vi "Get Named Ranges of Sheet.vi"(8 "error in":errorcluster, 10 "Sheet Name":string, 11 "SpreadsheetDocument":refnum<k24>) -> (0 "error out":errorcluster, 1 "Cells":string[][][](array[string]), 2 "Range Names":string[](array[string]), 3 "SpreadsheetDocument out":refnum<k24>)   [LabVIEW 2021, in "Open Xml.lvlib"]
uses:
  Open Xml.lvlib
  D:/git/Open-Xml-LabVIEW/Source/DocumentFormat.OpenXml.dll
  DocumentFormat.OpenXml.dll
  D:/git/Open-Xml-LabVIEW/Source/DocumentFormat.OpenXml.Framework.dll
  DocumentFormat.OpenXml.Framework.dll
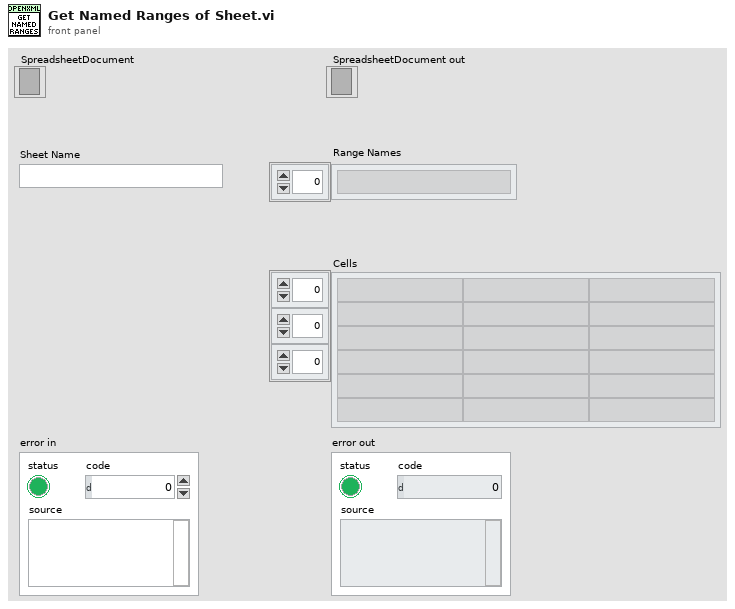
[diagram p1: front panel]
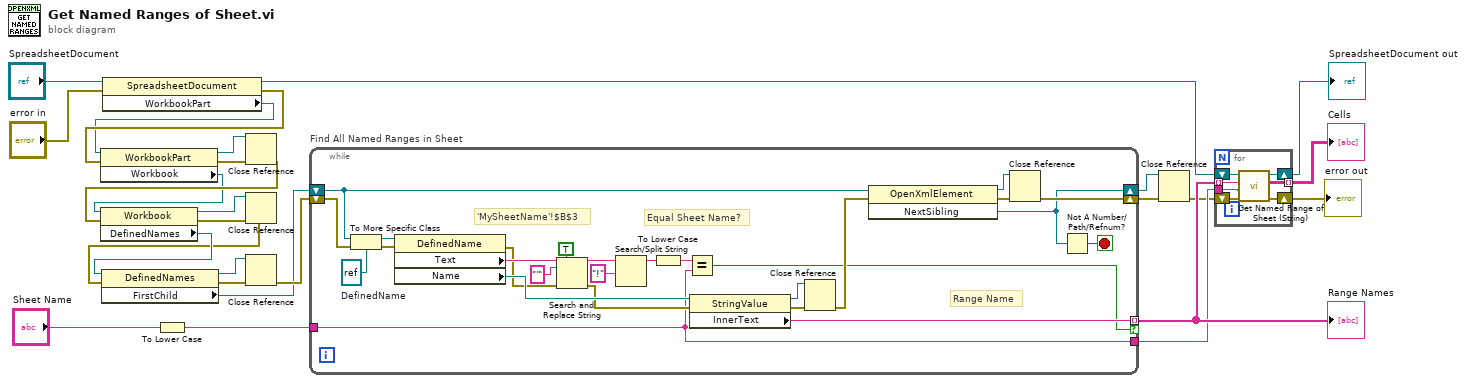
[diagram p0: block diagram]
diagram:
  n1 = property class="SpreadsheetDocument"(reference="SpreadsheetDocument", error in="error in") -> (reference out=w7:refnum<k24>, error out=w14:errorcluster, "WorkbookPart"=w13:refnum<k24>)
  n2 = property class="WorkbookPart"(reference=w13, error in=w14) -> (reference out=w23:refnum<k24>, error out=w25:errorcluster, "Workbook"=w11:refnum<k24>)
  n3 = To Lower Case(string="Sheet Name") -> (all lower case string=w1:string)
  n4 = Close Reference(reference=w23, error in (no error)=w25) -> (error out=w12:errorcluster)
  n5 = property class="Workbook"(reference=w11, error in=w12) -> (reference out=w21:refnum<k24>, error out=w24:errorcluster, "DefinedNames"=w27:refnum<k24>)
  n6 = Close Reference(reference=w21, error in (no error)=w24) -> (error out=w22:errorcluster)
  n7 = property class="DefinedNames"(reference=w27, error in=w22) -> (reference out=w20:refnum<k24>, error out=w26:errorcluster, "FirstChild"=w17:refnum<k24>)
  n8 = Close Reference(reference=w20, error in (no error)=w26) -> (error out=w18:errorcluster)
  n9 = while "Find All Named Ranges in Sheet" {
    shift-right: [w49] -> w9
    shift-left: w18 -> [w53]
    tunnel: w1 -> [w29]
    shift-right: [w44] -> w2
    shift-left: w17 -> [w45]
    tunnel: [w31] -> w10 mode=indexing if=w30
    tunnel: [w29] -> w6
    stop <- w52 stop-if-true
    w46 = refnum<k24> refnum  # DefinedName
    # "Equal Sheet Name?"
    # "'MySheetName'!$B$3"
    # "Range Name"
    n10 = To More Specific Class(target class=w46, reference=w45, error in=w53) -> (specific class reference=w51:refnum<k24>, error out=w50:errorcluster)
    n11 = property class="DefinedName"(reference=w51, error in=w50) -> (error out=w35:errorcluster, "Text"=w39:string, "Name"=w48:refnum<k24>)  [unwired: 1 out]
    n12 = Search and Replace String(replace all?=TRUE ("replace all? (F)"), input string=w39, search string="'", error in=w35) -> (result string=w41:string, error out=w34:errorcluster)  [unwired: 4 in, 2 out]
    n13 = Search/Split String(string=w41, search string/char (-)="!") -> (substring before match=w37:string)  [unwired: 1 in, 2 out]
    n14 = To Lower Case(string=w37) -> (all lower case string=w28:string)
    n15 = Equal?(x=w28, y=w29) -> (x = y?=w30:bool)
    n16 = property class="StringValue"(reference=w48, error in=w34) -> (reference out=w42:refnum<k24>, error out=w47:errorcluster, "InnerText"=w31:string)
    n17 = Close Reference(reference=w42, error in (no error)=w47) -> (error out=w43:errorcluster)
    n18 = invoke class="OpenXmlElement" method="NextSibling"(reference=w45, error in=w43) -> (reference out=w32:refnum<k24>, error out=w33:errorcluster, "NextSibling"=w44:refnum<k24>)  [unwired: 1 in]
    n19 = Close Reference(reference=w32, error in (no error)=w33) -> (error out=w49:errorcluster)
    n20 = Not A Number/Path/Refnum?(number/path/refnum=w44) -> (NaN/Path/Refnum?=w52:bool)
  }
  "Range Names" <- w10
  n21 = Close Reference(reference=w2, error in (no error)=w9) -> (error out=w3:errorcluster)
  n22 = for {
    tunnel: w10 -> [w60] mode=indexing
    shift-right: [w54] -> w8
    shift-left: w3 -> [w59]
    tunnel: w6 -> [w57]
    tunnel: [w56] -> w4 mode=indexing
    shift-right: [w55] -> w5
    shift-left: w7 -> [w58]
    n23 = call "Get Named Range of Sheet (String).vi"("error in"=w59, "Sheet Name"=w57, "Named Range Identifier"=w60, "SpreadsheetDocument"=w58) -> ("error out"=w54:errorcluster, "Cells"=w56:string[][], "SpreadsheetDocument out"=w55:refnum<k24>)  [unwired: 5 in]
  }
  "SpreadsheetDocument out" <- w5
  "error out" <- w8
  "Cells" <- w4
